vi "we1.vi"() -> (3 "Array 3":T1(array[cluster]))   [LabVIEW 2013]
uses:
  <vilib>/httpClient/LabVIEWHTTPClient.lvlib
panel:
  # "WEATHER REPORT"
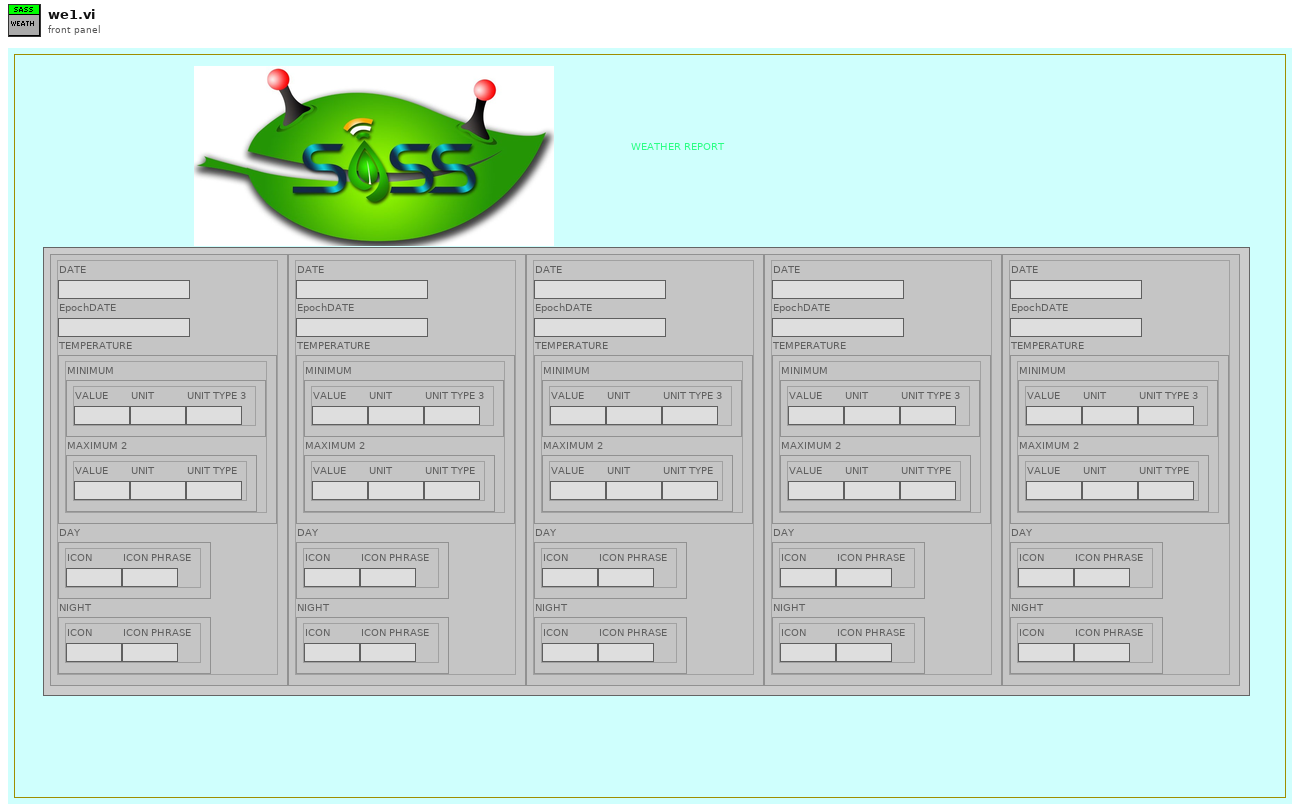
[diagram p1: front panel]
types:
  T1 = cluster{"DATE":string, "EpochDATE":string, "TEMPERATURE":cluster{"MINIMUM":cluster{"VALUE":string, "UNIT":string, "UNIT TYPE 3":string}, "MAXIMUM 2":cluster{"VALUE":string, "UNIT":string, "UNIT TYPE":string}}, "DAY ":cluster{"ICON":string, "ICON PHRASE":string}, "NIGHT":cluster{"ICON":string, "ICON PHRASE":string}}[]
  T2 = typedef "LabVIEWHTTPClient.lvlib/ClientHandle.ctl" = refnum<k1>
  T3 = cluster{"Date":string, "EpochDate":string, "Temperature":cluster{"Minimum":cluster{"Value":string, "Unit":string, "UnitType":string}, "Maximum":cluster{"Value":string, "Unit":string, "UnitType":string}}, "Day":cluster{"Icon":string, "IconPhrase":string}, "Night":cluster{"Icon":string, "IconPhrase":string}}[]
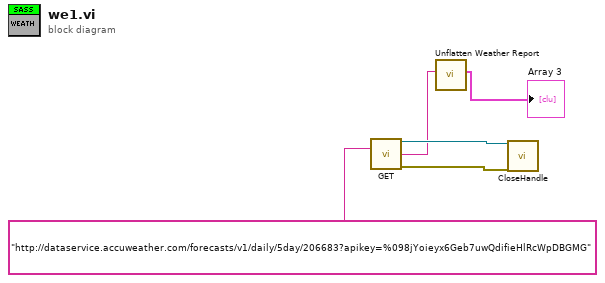
[diagram p0: block diagram]
diagram:
  n1 = call <vilib>:"GET.vi"("url"="http://dataservice.accuweather.com/forecasts/v1/daily/5day/206683?apikey=%098jYoieyx6Geb7uwQdifieHlRcWpDBGMG") -> ("client handle out"=w5:T2, "body"=w2:string, "error out"=w4:errorcluster)  [unwired: 11 in, 1 out]
  n2 = call "Unflatten Weather Report.vi"("String"=w2) -> ("Array"=→"Array 3":T3)  [unwired: 10 in]
  n3 = call <vilib>:"CloseHandle.vi"("client handle"=w5, "error in (no error)"=w4) -> ()  [unwired: 13 in, 1 out]
